vi "Subarray.vi"(8 "SamplesOffset":i32, 9 "I index":i32=3, 10 "Time":dbl[](array[numeric]), 11 "Synx":cdb[][](array[numeric])) -> (2 "Time subarray":dbl[](array[numeric]), 3 "Data subarray":cdb[][](array[numeric]))   [LabVIEW 2014, in "AppPlugins.lvlib" / "ModelValidationPlugin.lvclass"]
uses:
  ModelValidationPlugin.lvclass
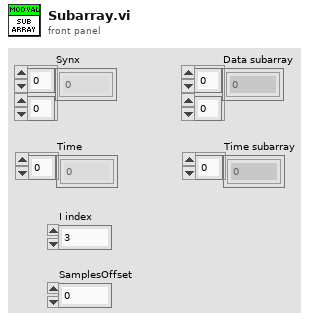
[diagram p1: front panel]
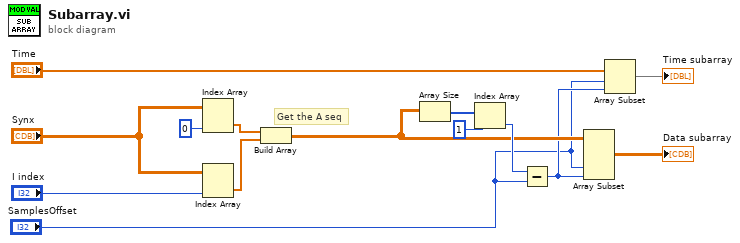
[diagram p0: block diagram]
diagram:
  # "Get the A seq"
  n1 = Index Array(array="Synx", index (col)=0 ("disabled index (col)")) -> (element=w7:cdb[])  [unwired: 1 in]
  n2 = Index Array(array="Synx", index (col)="I index") -> (element=w6:cdb[])  [unwired: 1 in]
  n3 = Build Array(w7, w6) -> (w5:cdb[][])
  n4 = Array Size(array=w5) -> (size(s)=w14:i32[])
  n5 = Index Array(array=w14, index=1) -> (element=w12:i32)
  n6 = Subtract(x=w12, y="SamplesOffset") -> (x-y=w2:i32)
  n7 = Array Subset(array=w5, index (col)="SamplesOffset", length (col)=w2) -> (→"Data subarray":cdb[][])  [unwired: 2 in]
  n8 = Array Subset(array="Time", index="SamplesOffset", length=w2) -> (→"Time subarray":dbl[])
